vi "WS7_setpoint.vi"(4 "tolerance":dbl=2e-06 format="%#_6e", 5 "lower (nm)":dbl=605.0, 6 "Stabilise":bool=TRUE, 7 "upper (nm)":dbl=740.0, 8 "error in (no error)":errorcluster, 9 "channel":i32=1, 10 "PID port":i32=1 min=1 max=2, 11 "set point":dbl=711.4636 caption="wavelength (nm)" format="%.2f") -> (0 "error out":errorcluster, 1 "rec wavelength (nm)":dbl=711.4636000140063, 2 "set point (out)":dbl)   [LabVIEW 2017]
uses:
  hardware/highfinesse/highfinesse.lvlib
panel:
  in  "max_attempts":i32=100
  out "attempts":i32
  out "err (nm)":dbl=4.2315184600738576e-07
  # "This vi sets the PID set point\nand reads back the measured \nwavelength on a given channel.\n\nPID loop should be configured \nin HighFinesse software (which\nmust be running)."
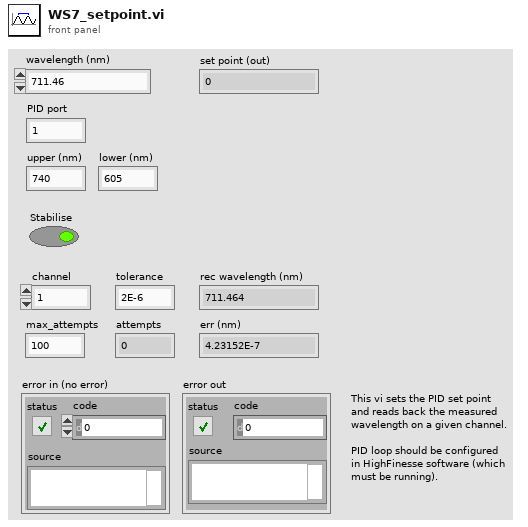
[diagram p1: front panel]
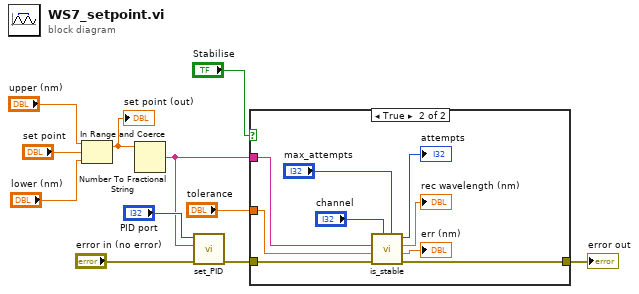
[diagram p0: block diagram]
diagram:
  n1 = In Range and Coerce(upper limit="upper (nm)", x="set point", lower limit="lower (nm)") -> (coerced(x)=w3:dbl)  [unwired: 1 out]
  "set point (out)" <- w3
  n2 = Number To Fractional String(number=w3) -> (F-format string=w1:string)  [unwired: 3 in]
  n3 = call "set_PID.vi"("error in (no error)"="error in (no error)", "wavelength (nm)"=w1, "port"="PID port") -> ("error out"=w6:errorcluster)  [unwired: 7 in, 1 out]
  n4 = case shown="True" "Stabilise" {
    tunnel: [w12 w21] -> w7
    tunnel: w6 -> [w12 w20]
    tunnel: "tolerance" -> [_ w19]
    tunnel: w1 -> [_ w17]
    frame False {
    }
    frame True {
      n5 = call "is_stable.vi"("max_attempts"="max_attempts", "ch"="channel", "error in (no error)"=w20, "tolerance"=w19, "set wavelength (nm)"=w17) -> ("error out"=w21:errorcluster, "err (nm)"=→"err (nm)":dbl, "rec wavelength (nm)"=→"rec wavelength (nm)":dbl, "attempts"=→"attempts":i32)  [unwired: 3 in]
    }
  }
  "error out" <- w7
